vi "To String (Object).vi"(0 "Variant in":variant, 5 "indent":i32, 7 "enable LabVIEW extensions? (T)":bool=TRUE, 9 "pretty print? (T)":bool=TRUE, 11 "error in (no error)":errorcluster) -> (4 "String":string, 15 "error out":errorcluster)   [LabVIEW 2017, in "Advanced Variant Tools.lvlib"]
doc: "Flattens the given JSON data to a string."
uses:
  Advanced Variant Tools.lvlib
  Variant Data Manipulation/Source/Variant Data Manipulation.lvlib
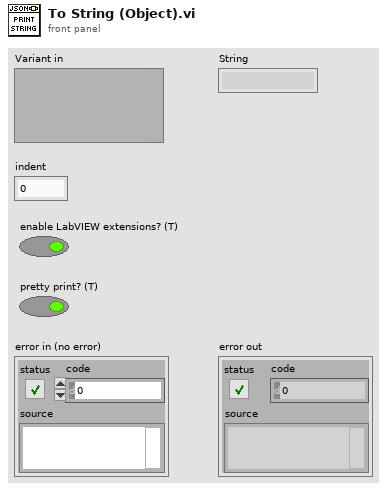
[diagram p1: front panel]
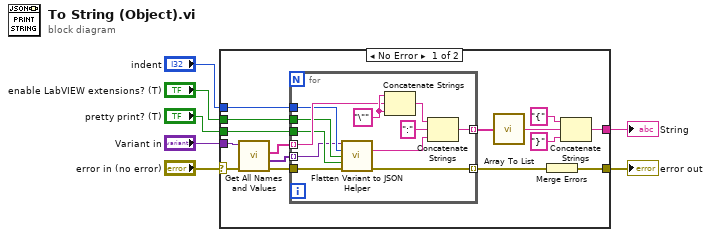
[diagram p0: block diagram]
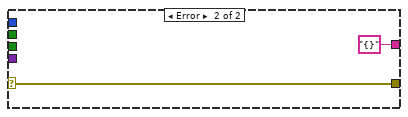
[diagram p2: hidden frame]
diagram:
  n1 = case shown="No Error" "error in (no error)" {
    selector: "error in (no error)" -> [w11 w35]
    tunnel: "Variant in" -> [w12 _]
    tunnel: [w22 "{}"] -> w6
    tunnel: [w18 w35] -> w4
    tunnel: "enable LabVIEW extensions? (T)" -> [w15 _]
    tunnel: "indent" -> [w14 _]
    tunnel: "pretty print? (T)" -> [w10 _]
    frame No Error {
      n2 = call "Get All Names and Values.vi"("error in"=w11, "Cluster in"=w12) -> ("error out"=w9:errorcluster, "Values"=w8:variant[], "Element Names"=w13:string[])  [unwired: 5 in, 2 out]
      n3 = for {
        tunnel: w13 -> [w31] mode=indexing
        tunnel: w8 -> [w24] mode=indexing
        tunnel: [w33] -> w21 mode=indexing
        tunnel: w9 -> [w25]
        tunnel: [w29] -> w19 mode=indexing
        tunnel: w15 -> [w28]
        tunnel: w14 -> [w27]
        tunnel: w10 -> [w26]
        w32 = "\"" ("string")
        n4 = call "Flatten Variant to JSON Helper.vi"("Variant in"=w24, "indent"=w27, "enable LabVIEW extensions? (T)"=w28, "pretty print? (T)"=w26, "error in (no error)"=w25) -> ("String"=w23:string, "error out"=w29:errorcluster)  [unwired: 8 in, 1 out]
        n5 = Concatenate Strings(w32, w31, w32) -> (w30:string)
        n6 = Concatenate Strings(w30, ":" ("string"), w23) -> (w33:string)
      }
      n7 = call "Array To List.vi"("Array"=w21) -> ("String"=w20:string)  [unwired: 14 in]
      n8 = Merge Errors(w19) -> (w18:errorcluster)
      n9 = Concatenate Strings("{" ("string"), w20, "}" ("string")) -> (w22:string)
    }
    frame Error {
    }
  }
  "String" <- w6
  "error out" <- w4
